vi "LEIN reply pack out if ACTI 6.vi"(7 "LEIN reply holder":T2={"Reply msg(cmdif no reply)"={"SID"=0, "ANF"=FALSE, "CMD"=enum."TASK", "DATA"=[]}, "Reply time"=timestamp(0 s since 1904-01-01), "Valid reply"=FALSE}, 11 "error in (no error)":errorcluster) -> (2 "CMD":T1, 3 "Valid reply":bool, 4 "ANF":bool, 6 "SID":u8, 8 "Reply(CMD if no reply)":T3, 15 "error out":errorcluster)   [LabVIEW 2011]
uses:
  Defenitions/LEIN CMD Cluster.ctl
  Defenitions/LEIN CMD List.ctl
  Defenitions/LEIN Reply Holder.ctl
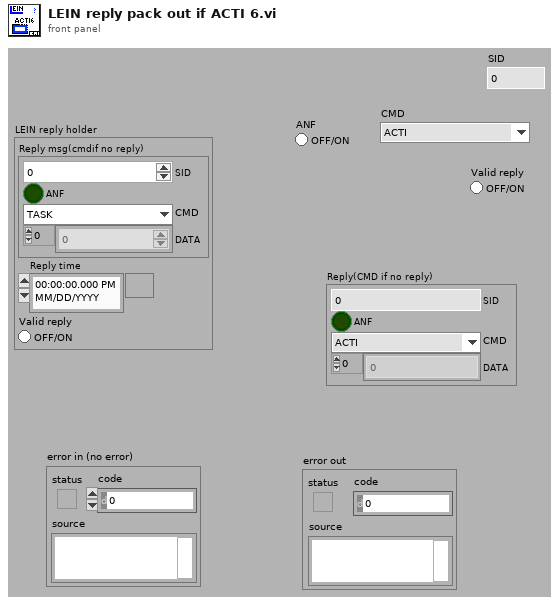
[diagram p1: front panel]
types:
  T1 = typedef "LEIN CMD List.ctl" = enum8{"ACTI", "TASK", "RES0", "STAT", "RES1", "RES2", "RES3", "USER"}
  T2 = typedef "LEIN Reply Holder.ctl" = cluster{"Reply msg(cmdif no reply)":T3, "Reply time":timestamp, "Valid reply":bool}
  T3 = typedef "LEIN CMD Cluster.ctl" = cluster{"SID":u8, "ANF":bool, "CMD":T1, "DATA":u8[]}
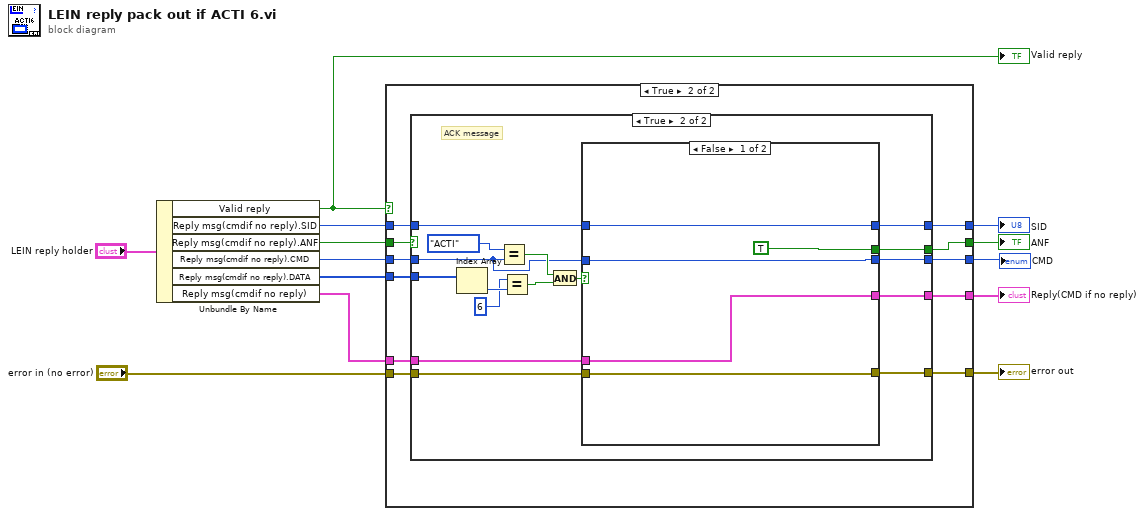
[diagram p0: block diagram]
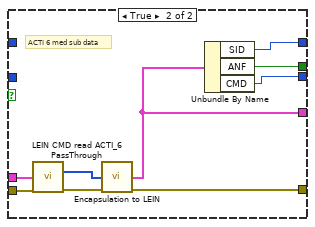
[diagram p4: hidden frame]
diagram:
  n1 = Unbundle By Name("LEIN reply holder") -> ("Valid reply"=w2:bool, "Reply msg(cmdif no reply).SID"=w5:u8, "Reply msg(cmdif no reply).ANF"=w9:bool, "Reply msg(cmdif no reply).CMD"=w6:T1, "Reply msg(cmdif no reply).DATA"=w7:u8[], "Reply msg(cmdif no reply)"=w8:T3)
  "Valid reply" <- w2
  n2 = case shown="True" w2 {
    tunnel: [w17 w29] -> w13
    tunnel: [w15 w28] -> w12
    tunnel: [w16 w27] -> w11
    tunnel: "error in (no error)" -> [w16 w26]
    tunnel: w9 -> [w17 w25]
    tunnel: w8 -> [w15 w24]
    tunnel: w7 -> [_ w23]
    tunnel: w6 -> [w14 w22]
    tunnel: w5 -> [w18 w21]
    tunnel: [w18 w20] -> w4
    tunnel: [w14 w19] -> w1
    frame False {
    }
    frame True {
      n3 = case shown="True" w25 {
        selector: w25 -> [w34 _]
        tunnel: w22 -> [w30 w35]
        tunnel: w23 -> [_ w50]
        tunnel: w24 -> [w31 w43]
        tunnel: w26 -> [w33 w42]
        tunnel: [w33 w41] -> w27
        tunnel: [w31 w40] -> w28
        tunnel: [w34 w39] -> w29
        tunnel: w21 -> [w32 w38]
        tunnel: [w32 w37] -> w20
        tunnel: [w30 w36] -> w19
        frame False {
        }
        frame True {
          # "ACK message"
          n4 = Index Array(array=w50) -> (element=w49:u8)  [unwired: 1 in]
          n5 = Equal?(x=LEIN_CMD_List."ACTI", y=w35) -> (x = y?=w46:bool)
          n6 = Equal?(x=u8 6, y=w49) -> (x = y?=w45:bool)
          n7 = And(x=w46, y=w45) -> (x .and. y?=w44:bool)
          n8 = case shown="False" w44 {
            tunnel: w43 -> [w54 w64]
            tunnel: w42 -> [w55 w61]
            tunnel: [w55 w57] -> w41
            tunnel: [w54 w58] -> w40
            tunnel: [TRUE ("ANF") w60] -> w39
            tunnel: w38 -> [w52 _]
            tunnel: [w52 w59] -> w37
            tunnel: [w51 w56] -> w36
            tunnel: w35 -> [w51 _]
            frame False {
            }
            frame True {
              # "ACTI 6 med sub data"
              n9 = call "LEIN CMD read ACTI_6 PassThrough.vi"("CMD"=w64, "error in (no error)"=w61) -> ("Reply from sub ID"=w63:u8[], "error out"=w62:errorcluster)  [unwired: 10 in, 2 out]
              n10 = call "Encapsulation to LEIN.vi"("Data and header"=w63, "error in (no error)"=w62) -> ("CMD out"=w58:T3, "error out"=w57:errorcluster)  [unwired: 10 in, 2 out]
              n11 = Unbundle By Name(w58) -> ("SID"=w59:u8, "ANF"=w60:bool, "CMD"=w56:T1)
            }
          }
        }
      }
    }
  }
  "ANF" <- w13
  "Reply(CMD if no reply)" <- w12
  "error out" <- w11
  "SID" <- w4
  "CMD" <- w1
